vi "LEBITVacuum.ReadDbase.vi"(0 "i ref in":refnum<vi>, 2 "Data Source":string="LBADD", 5 "error in (no error)":errorcluster, 9 "Associated Panels":string[](array[string])=["Buncher", "TestIonSource", "Penning", "BuntoPenning", "PenningEject", "Mcp&PhosVol", "GasCell", "IonGuide", "N4toBob1", "Bob1toBun"]) -> (14 "i ref out":refnum<vi>, 16 "DBArray":string[][](array[string]), 17 "Safety Array":string[][](array[string]), 18 "Ambient Measurements":string[][](array[string]), 19 "error out":errorcluster)   [LabVIEW 2014, in "LEBITVacuum.lvlib"]
uses:
  LEBITVacuum.lvlib
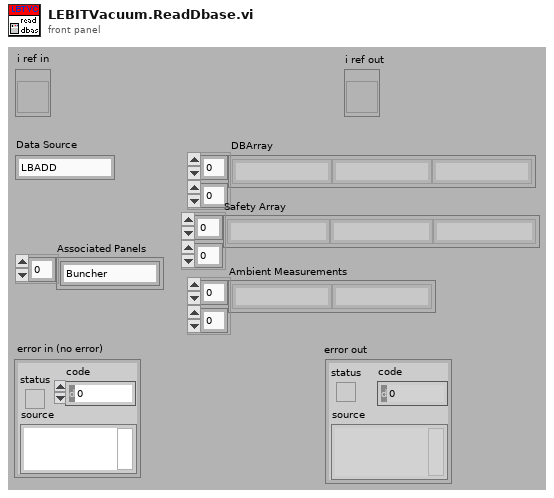
[diagram p1: front panel]
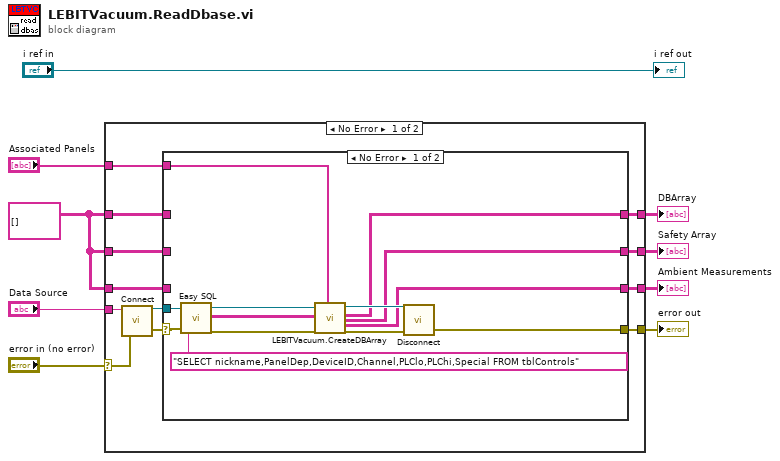
[diagram p0: block diagram]
diagram:
  w3 = string[][] [] ("DBArrayIn")
  n1 = case shown="No Error" "error in (no error)" {
    selector: "error in (no error)" -> [w20 w42]
    tunnel: "Data Source" -> [w21 _]
    tunnel: [w17 w42] -> w6
    tunnel: w3 -> [w16 w41]
    tunnel: [w15 w41] -> w8
    tunnel: [w14 w40] -> w4
    tunnel: w3 -> [w13 w40]
    tunnel: [w12 w39] -> w2
    tunnel: w3 -> [w11 w39]
    tunnel: "Associated Panels" -> [w10 _]
    frame No Error {
      n2 = call <vilib>:"Connect.vi"("error in (no error)"=w20, "data source name"=w21) -> ("error out"=w18:errorcluster, "Connection"=w19:refnum<k7>)  [unwired: 2 in]
      n3 = case shown="No Error" w18 {
        selector: w18 -> [w26 w38]
        tunnel: w19 -> [w28 _]
        tunnel: [w29 w38] -> w17
        tunnel: w16 -> [_ w37]
        tunnel: [w25 w37] -> w15
        tunnel: [w24 w36] -> w14
        tunnel: w13 -> [_ w36]
        tunnel: [w23 w35] -> w12
        tunnel: w11 -> [_ w35]
        tunnel: w10 -> [w22 _]
        frame No Error {
          n4 = call <vilib>:"Easy SQL.vi"("connection"=w28, "SQL statement"="SELECT nickname,PanelDep,DeviceID,Channel,PLClo,PLChi,Special FROM tblControls", "error in (no error)"=w26) -> ("connection"=w30:refnum<k7>, "error out"=w32:errorcluster, "query results"=w27:string[][])  [unwired: 2 out]
          n5 = call "LEBITVacuum.CreateDBArray.vi"("connection in"=w30, "query results"=w27, "error in"=w32, "Associated Panels"=w22) -> ("connection out"=w33:refnum<k7>, "DBArray"=w25:string[][], "Safety Array"=w24:string[][], "Ambient Measurements"=w23:string[][], "error out"=w31:errorcluster)  [unwired: 11 in]
          n6 = call <vilib>:"Disconnect.vi"("error in (no error)"=w31, "connection"=w33) -> ("error out"=w29:errorcluster)  [unwired: 1 in]
        }
        frame Error {
        }
      }
    }
    frame Error {
      (unwired) 0
    }
  }
  "error out" <- w6
  "DBArray" <- w8
  "Safety Array" <- w4
  "Ambient Measurements" <- w2
  "i ref out" <- "i ref in"
